vi "Test Oxford ITC 503.vi"() -> ()   [LabVIEW 2016]
panel:
  out "after flush":errorcluster
  in  "Flush buffer":bool
  in  "write buffer":string="C1"
  in  "Test read chan":bool
  out "VISA resource name out":refnum<visa-resource-name>
  out "Data":dbl
  out "read buffer 2":string
  in  "Channel #":i32=1
  out "status byte":u16 format="%b"
  out "read buffer":string[](array[string])
  in  "milliseconds to wait":u32=500
  in  "VISA resource name":refnum<visa-resource-name>
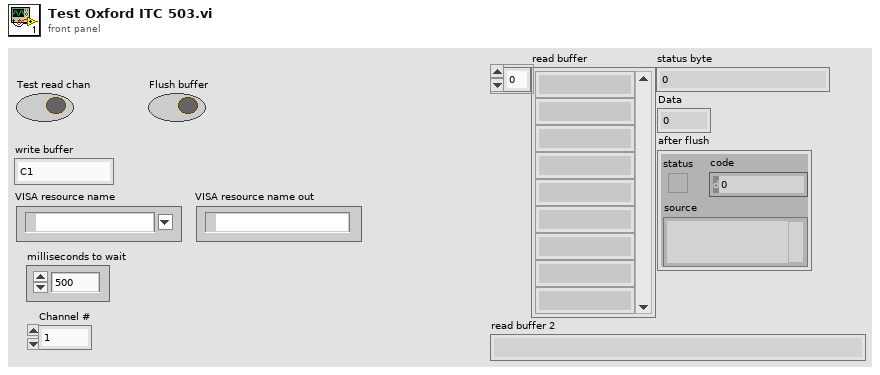
[diagram p1: front panel]
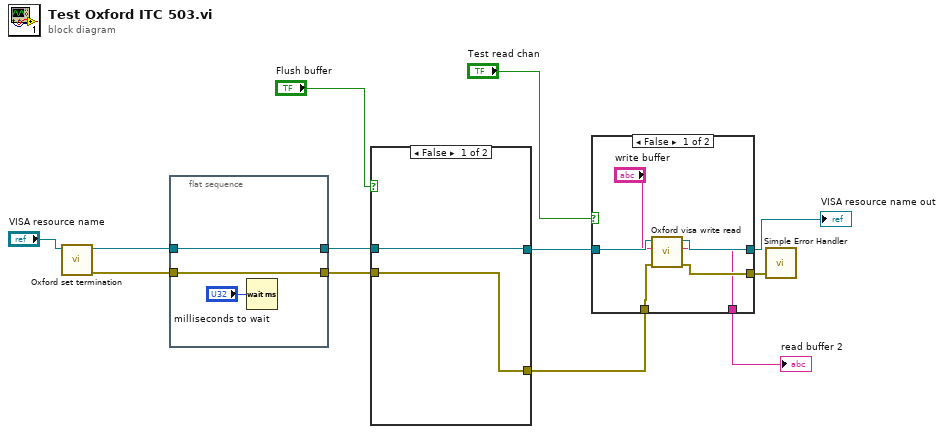
[diagram p0: block diagram]
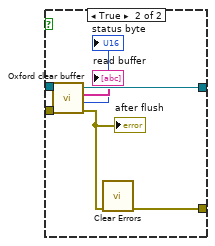
[diagram p2: hidden frame]
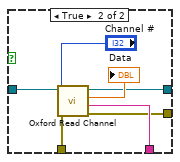
[diagram p3: hidden frame]
diagram:
  n1 = call "Oxford set termination.vi"("VISA resource name"="VISA resource name") -> ("error out"=w11:errorcluster, "VISA resource name out"=w10:refnum<visa-resource-name>)  [unwired: 9 in]
  n2 = flat-sequence {
    tunnel: w11 -> [w14]
    tunnel: [w14] -> w9
    tunnel: w10 -> [w13]
    tunnel: [w13] -> w8
    frame #0 {
      n3 = Wait (ms)(milliseconds to wait="milliseconds to wait") -> ()  [unwired: 1 out]
    }
  }
  n4 = case shown="False" "Flush buffer" {
    tunnel: w9 -> [w16 w24]
    tunnel: w8 -> [w17 w23]
    tunnel: [w17 w22] -> w7
    tunnel: [w16 w21] -> w3
    frame False {
    }
    frame True {
      n5 = call "Oxford clear buffer.vi"("error in (no error)"=w24, "VISA resource name"=w23) -> ("error out"=w20:errorcluster, "status byte"=→"status byte":u16, "read buffer"=→"read buffer":string[], "VISA resource name out"=w22:refnum<visa-resource-name>)  [unwired: 6 in]
      "after flush" <- w20
      n6 = call <vilib>:"Clear Errors.vi"("error in (no error)"=w20) -> ("error out"=w21:errorcluster)  [unwired: 5 in, 1 out]
    }
  }
  n7 = case shown="False" "Test read chan" {
    tunnel: w7 -> [w30 w37]
    tunnel: [w25 w35] -> w6
    tunnel: [w28 w33] -> w5
    tunnel: [w27 w32] -> w4
    tunnel: w3 -> [w29 w31]
    frame False {
      n8 = call "Oxford visa write read.vi"("error in (no error)"=w29, "write buffer"="write buffer", "VISA resource name"=w30) -> ("error out"=w28:errorcluster, "read buffer"=w25:string, "VISA resource name out"=w27:refnum<visa-resource-name>)  [unwired: 6 in]
    }
    frame True {
      n9 = call "Oxford Read Channel.vi"("error in (no error)"=w31, "Channel #"="Channel #", "VISA resource name"=w37) -> ("error out"=w33:errorcluster, "read buffer"=w35:string, "Data"=→"Data":dbl, "VISA resource name out"=w32:refnum<visa-resource-name>)  [unwired: 5 in]
    }
  }
  "read buffer 2" <- w6
  "VISA resource name out" <- w4
  n10 = call <vilib>:"Simple Error Handler.vi"("error in (no error)"=w5) -> ()  [unwired: 4 in, 5 out]
